vi "Loggen FTIR.vi"   [LabVIEW 2020, in "LogKonfig.lvlib"]
uses:
  LogKonfig.lvlib
  FT-IR/FGV FT-IR Aktionen.ctl
  FT-IR/FT-IR.lvlib
types:
  T1 = typedef "FT-IR.lvlib/FGV FT-IR Aktionen.ctl" = enum16{"lesen", "NOG setzen", "NOS setzen", "Initialisieren", "speichern", "ALLES setzen", "FT-IR Spektrum loggen", "Komm Stoppen", "Spektrum LogKonfig"}
  T2 = cluster{"(80) labEnabled":bool, "(81) labPath":path, "(82) labBaseName":string, "(83) labIndex":string, "Spektrum loggen aktiv?":bool}
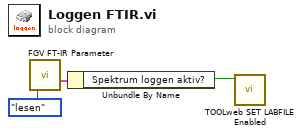
[diagram p0: block diagram]
diagram:
  n1 = call "FGV FT-IR Parameter.vi"("Aktion"=FGV_FT-IR_Aktionen."lesen") -> ("Ausgangs-Cluster"=w3:T2)  [unwired: 11 in, 7 out]
  n2 = Unbundle By Name(w3) -> ("Spektrum loggen aktiv?"=w1:bool)
  n3 = call "TOOLweb SET LABFILE Enabled.vi"("Enabled"=w1) -> ()  [unwired: 2 in, 5 out]
